vi "Read_date_time_string.vi"(10 "Time":string, 11 "Date (or Date_time)":string) -> (1 "Y/M/D/H/M/S":dbl[](array[numeric]), 2 "time in seconds":dbl format="%.6f", 3 "time stamp":timestamp, 5 "date time record":T1)   [LabVIEW 2016]
uses:
  <vilib>/Utility/miscctls.llb/LVDateTimeRec.ctl
  <vilib>/Utility/error.llb/whitespace.ctl
panel:
  out "date time rec":T1
  out "offset past match Date/Tine":i32
  out "offset past match  AM/PM":i32
  out "hour":dbl
  out "minutes":dbl
  out "seconds":dbl
  out "Year":dbl
  out "day of month":dbl
  out "month":dbl
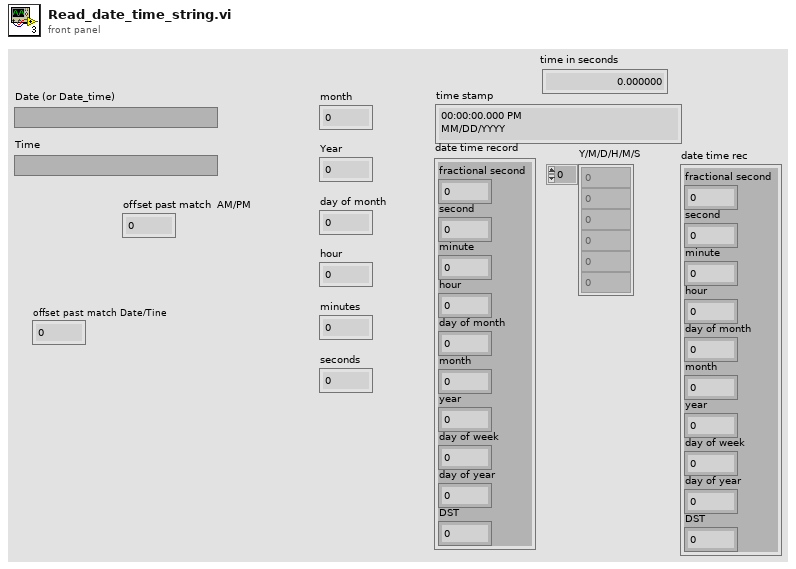
[diagram p1: front panel]
types:
  T1 = typedef "LVDateTimeRec.ctl" = cluster{"fractional second":dbl, "second":i32, "minute":i32, "hour":i32, "day of month":i32, "month":i32, "year":i32, "day of week":i32, "day of year":i32, "DST":i32}
  T2 = typedef "whitespace.ctl" = u16
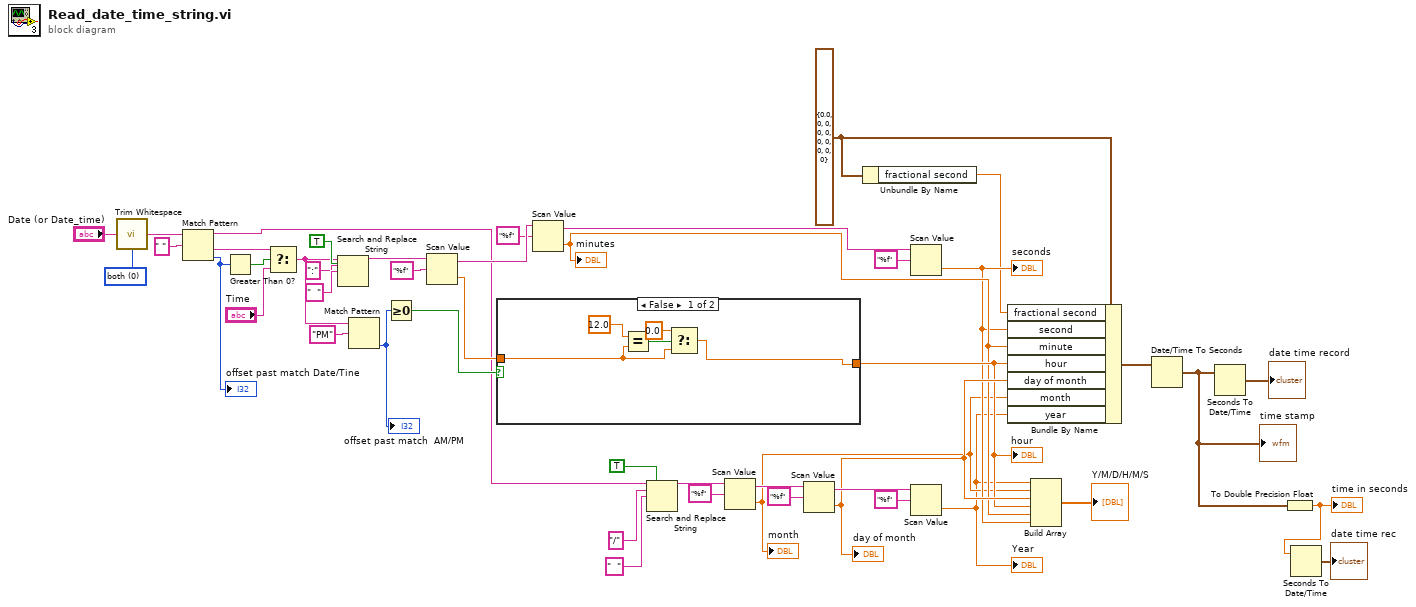
[diagram p0: block diagram]
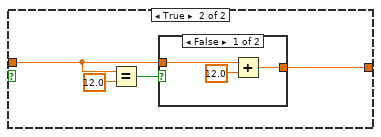
[diagram p2: hidden frame]
diagram:
  w8 = T2 0 items=["both", "start of string", "end of string"] ("location (both)")
  w16 = T1 {"fractional second"=0.0, "second"=0, "minute"=0, "hour"=0, "day of month"=0, "month"=0, "year"=0, "day of week"=0, "day of year"=0, "DST"=0}
  n1 = call <vilib>:"Trim Whitespace.vi"("string"="Date (or Date_time)", "location (both)"=w8) -> ("trimmed string"=w9:string)
  n2 = Match Pattern(string=w9, regular expression=" ") -> (before substring=w11:string, after substring=w5:string, offset past match=w7:i32)  [unwired: 1 in, 1 out]
  "offset past match Date/Tine" <- w7
  n3 = Greater Than 0?(x=w7) -> (x > 0?=w6:bool)
  n4 = Select(t=w5, s=w6, f="Time") -> (s? t:f=w3:string)
  n5 = Search and Replace String(replace all?=TRUE ("replace all? (F)"), input string=w3, search string=":", replace string="  " ("replace string (\"\")")) -> (result string=w35:string)  [unwired: 4 in, 3 out]
  n6 = Match Pattern(string=w3, regular expression="PM") -> (offset past match=w27:i32)  [unwired: 1 in, 3 out]
  "offset past match  AM/PM" <- w27
  n7 = Greater Or Equal To 0?(x=w27) -> (x >= 0?=w26:bool)
  n8 = Scan Value(string=w35, format string="%f") -> (output string=w31:string, value=w25:dbl)  [unwired: 1 in]
  n9 = case shown="False" w26 {
    tunnel: w25 -> [w48 w53]
    tunnel: [w47 w55] -> w23
    frame False {
      n10 = Equal?(x=12.0 ("y"), y=w48) -> (x = y?=w51:bool)
      n11 = Select(t=0.0, s=w51, f=w48) -> (s? t:f=w47:dbl)
    }
    frame True {
      n12 = Equal?(x=w53, y=12.0) -> (x = y?=w54:bool)
      n13 = case shown="False" w54 {
        tunnel: w53 -> [w58 w59]
        tunnel: [w56 w59] -> w55
        frame False {
          n14 = Add(x=w58, y=12.0) -> (x+y=w56:dbl)
        }
        frame True {
        }
      }
    }
  }
  "hour" <- w23
  n15 = Scan Value(string=w31, format string="%f") -> (output string=w37:string, value=w22:dbl)  [unwired: 1 in]
  "minutes" <- w22
  n16 = Search and Replace String(replace all?=TRUE ("replace all? (F)"), input string=w11, search string="/", replace string="  " ("replace string (\"\")")) -> (result string=w40:string)  [unwired: 4 in, 3 out]
  n17 = Scan Value(string=w40, format string="%f") -> (output string=w44:string, value=w18:dbl)  [unwired: 1 in]
  "month" <- w18
  n18 = Scan Value(string=w44, format string="%f") -> (output string=w38:string, value=w24:dbl)  [unwired: 1 in]
  "day of month" <- w24
  n19 = Unbundle By Name(w16) -> ("fractional second"=w19:dbl)
  n20 = Scan Value(string=w37, format string="%f") -> (value=w21:dbl)  [unwired: 1 in, 1 out]
  "seconds" <- w21
  n21 = Scan Value(string=w38, format string="%f") -> (value=w17:dbl)  [unwired: 1 in, 1 out]
  "Year" <- w17
  n22 = Bundle By Name(cluster=w16, "fractional second"=w19, "second"=w21, "minute"=w22, "hour"=w23, "day of month"=w24, "month"=w18, "year"=w17) -> (w15:T1)
  n23 = Build Array(w17, w18, w24, w23, w22, w21) -> (→"Y/M/D/H/M/S":dbl[])
  n24 = Date/Time To Seconds(2:w15) -> (0:w14:timestamp)  [unwired: 1 in]
  "time stamp" <- w14
  n25 = Seconds To Date/Time(time stamp (now)=w14) -> (date time rec=→"date time record":T1)  [unwired: 1 in]
  n26 = To Double Precision Float(number=w14) -> (double precision float=w2:dbl)
  "time in seconds" <- w2
  n27 = Seconds To Date/Time(time stamp (now)=w2) -> (date time rec=→"date time rec":T1)  [unwired: 1 in]
